vi "reset.vi"(0 "NInstrSim":refnum<class "NInstrSim.lvclass">, 5 "error in (no error)":errorcluster) -> (14 "dup NInstrSim":refnum<class "NInstrSim.lvclass">, 19 "error out":errorcluster)   [LabVIEW 2009, in "HB_Device_Examples.lvlib" / "NInstrSim.lvclass"]
doc: "This VI resets the instrument, and then sends a set of default setup commands to the instrument."
uses:
  NInstrSim.lvclass
  lib.lib/HGF_LVC/HGF_DeviceBaseClasses/HGF_VISADevice/HGF_VISADevice.lvclass
  non_GPL/instr.lib/NI Instrument Simulator/NI Instrument Simulator.lvlib
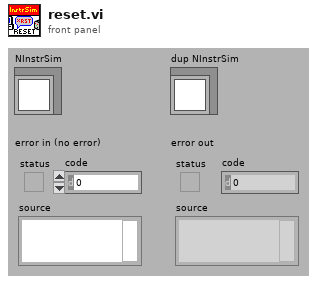
[diagram p1: front panel]
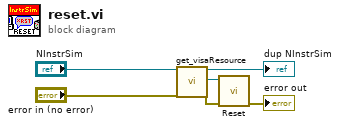
[diagram p0: block diagram]
diagram:
  n1 = call "get_visaResource.vi"("HGF_VISADevice"="NInstrSim", "error in (no error)"="error in (no error)") -> ("dup HGF_VISADevice"=→"dup NInstrSim":refnum<class "NInstrSim.lvclass">, "VISA Resource Name"=w5:refnum<visa-resource-name>, "error out"=w4:errorcluster)  [unwired: 15 out]
  n2 = call "Reset.vi"("error in (no error)"=w4, "VISA resource name"=w5) -> ("error out"=→"error out":errorcluster)  [unwired: 9 out]
